vi "query_UIM_ICFG.vi"(8 "error in (no error)":errorcluster caption="错误输入（无错误）", 11 "StepMotor输入":refnum<class "StepMotor.lvclass">) -> (0 "error out":errorcluster caption="错误输出", 2 "ICFG输入":T1, 3 "StepMotor输出":refnum<class "StepMotor.lvclass">)   [LabVIEW 2016, in "MotionControl.lvlib" / "StepMotor.lvclass"]
uses:
  <userlib>/MotionControl/StepMotor/StepMotor.lvclass
  <userlib>/MotionControl/StepMotor/StepMotor.lvclass/StepMotor.ctl
  <userlib>/UISimCanFunc_wrapper/UISimCanFunc_wrapper.lvlib
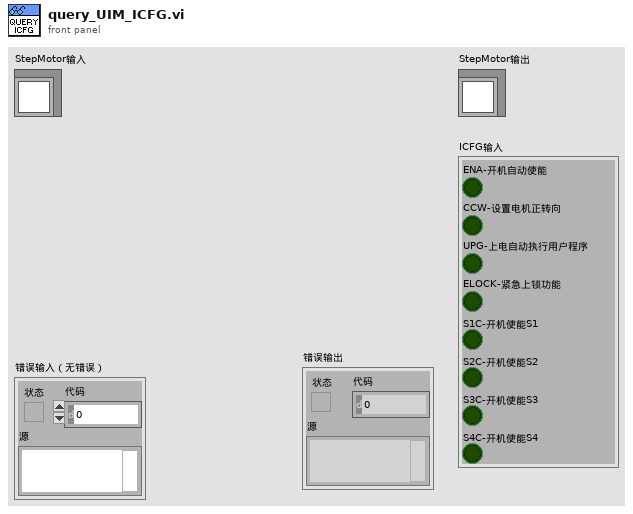
[diagram p1: front panel]
types:
  T1 = cluster{"ENA-开机自动使能":bool, "CCW-设置电机正转向":bool, "UPG-上电自动执行用户程序":bool, "ELOCK-紧急上锁功能":bool, "S1C-开机使能S1":bool, "S2C-开机使能S2":bool, "S3C-开机使能S3":bool, "S4C-开机使能S4":bool}
  T2 = typedef "UISimCanFunc_wrapper.lvlib/UIM_ICFG_INFO_OBJ.ctl" = cluster{"bENA":bool, "bCCW":bool, "bPROG":bool, "bELOCK":bool, "bS1C":bool, "bS2C":bool, "bS3C":bool, "bP4C":bool}
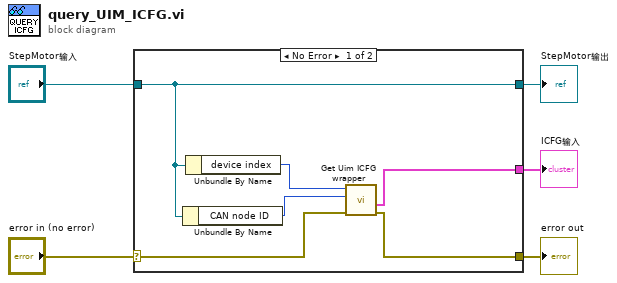
[diagram p0: block diagram]
diagram:
  n1 = case shown="No Error" "error in (no error)" {
    selector: "error in (no error)" -> [w8 w12]
    tunnel: [w7 w12] -> w4
    tunnel: [w11 w13] -> w2
    tunnel: "StepMotor输入" -> [w11 w13]
    tunnel: [w6 _] -> w1
    frame No Error {
      n2 = Unbundle By Name(w11) -> ("CAN node ID"=w9:u32)
      n3 = Unbundle By Name(w11) -> ("device index"=w10:u32)
      n4 = call <userlib>:"Get Uim ICFG wrapper.vi"("error in (no error)"=w8, "dwCanNodeId"=w9, "dwDevIndex"=w10) -> ("error out"=w7:errorcluster, "UIM_ICFG_INFO_OBJ"=w6:T2)  [unwired: 6 in, 1 out]
    }
    frame Error {
    }
  }
  "error out" <- w4
  "StepMotor输出" <- w2
  "ICFG输入" <- w1
